vi "Settings Dialog.vi"(0 "Settings in":T9 {"Processing Settings"."Test Parameters"."Allowed Tolerance (%) FS" format="%#_4g"; "Acq Settings"."Config Settings"."Simulated Sensor Injection" scale=0.0..100.0}, 1 "Database in":refnum<queue>, 11 "error in (no error)":errorcluster) -> (3 "Database out":refnum<queue>, 4 "Settings out":T9 {"Processing Settings"."Test Parameters"."Allowed Tolerance (%) FS" format="%#_4g"; "Acq Settings"."Config Settings"."Simulated Sensor Injection" scale=0.0..100.0}, 6 "Measurements out":T7[](array[typedef]), 8 "UI Refresh Needed?":bool, 10 "Cancelled?":bool, 15 "error out":errorcluster)   [LabVIEW 2026, in "Settings.lvlib"]
doc: "Dialog for selecting user specified settings."
uses:
  Settings.lvlib
  controls/UI/Settings Cluster.ctl
  controls/UI/Acq Settings.ctl
  Acquisition/Instrument Specifications Configuration.ctl
  Acquisition/Instrument Specifications Cluster Configuration.ctl
  controls/UI/Measurement Role.ctl
  controls/UI/Config Settings.ctl
  Processing/Processing Settings.ctl
  controls/Messaging Payloads/Sensor CoreData.ctl
  controls/Messaging Payloads/Sensor CoreData Cluster.ctl
  controls/UI/Units Enum.ctl
  controls/UI/Signal Enum.ctl
  Processing/Test Parameters.ctl
  Processing/Test Parameters Cluster.ctl
  controls/UI/Test Sequence Context.ctl
  controls/UI/Direction.ctl
  controls/UI/Session Identfiers.ctl
  controls/UI/Test Sequence Settings.ctl
  controls/UI/Test Sequence State.ctl
  controls/UI/Test Sequence Enum.ctl
  controls/Controller/Stimulus Settings.ctl
  controls/Controller/Stimulus Outputs.ctl
  controls/Controller/Stimulus Output.ctl
  controls/Controller/Controller Core Data.ctl
  controls/Controller/Stimulus Output Configuration.ctl
  controls/Controller/Stimulus Role.ctl
  support/Architecture/Message Queue/Message Cluster.ctl
  controls/UI/Measurements Config.ctl
  controls/UI/Measurement Config.ctl
  controls/UI/Stimulus Outputs Display.ctl
  controls/UI/Stimulus Output Display.ctl
  controls/UI/Settings Refs.ctl
  controls/UI/UI List Type.ctl
  controls/UI/Data Entity.ctl
  Acquisition/Acquisition.lvlib
  support/Architecture/Message Queue/Message Queue.lvlib
  Processing/Processing_Engine.lvlib
panel:
  in  "STIMULUS OUTPUTS":T1
  out "INSTRUMENT CONFIGURATIONS":T4
  in  "MEASUREMENTS":T8
  in  "Operator":string(combo)
  in  "Cancel Button":bool
  in  "OK Button":bool
  # "Non visible portion of dialog (needed for connector pane)."
  # "* Database-configured values. Maintained by an Administrator."
  # "Physical Channel and Measurement Role are assigned in the Measurements section directly below."
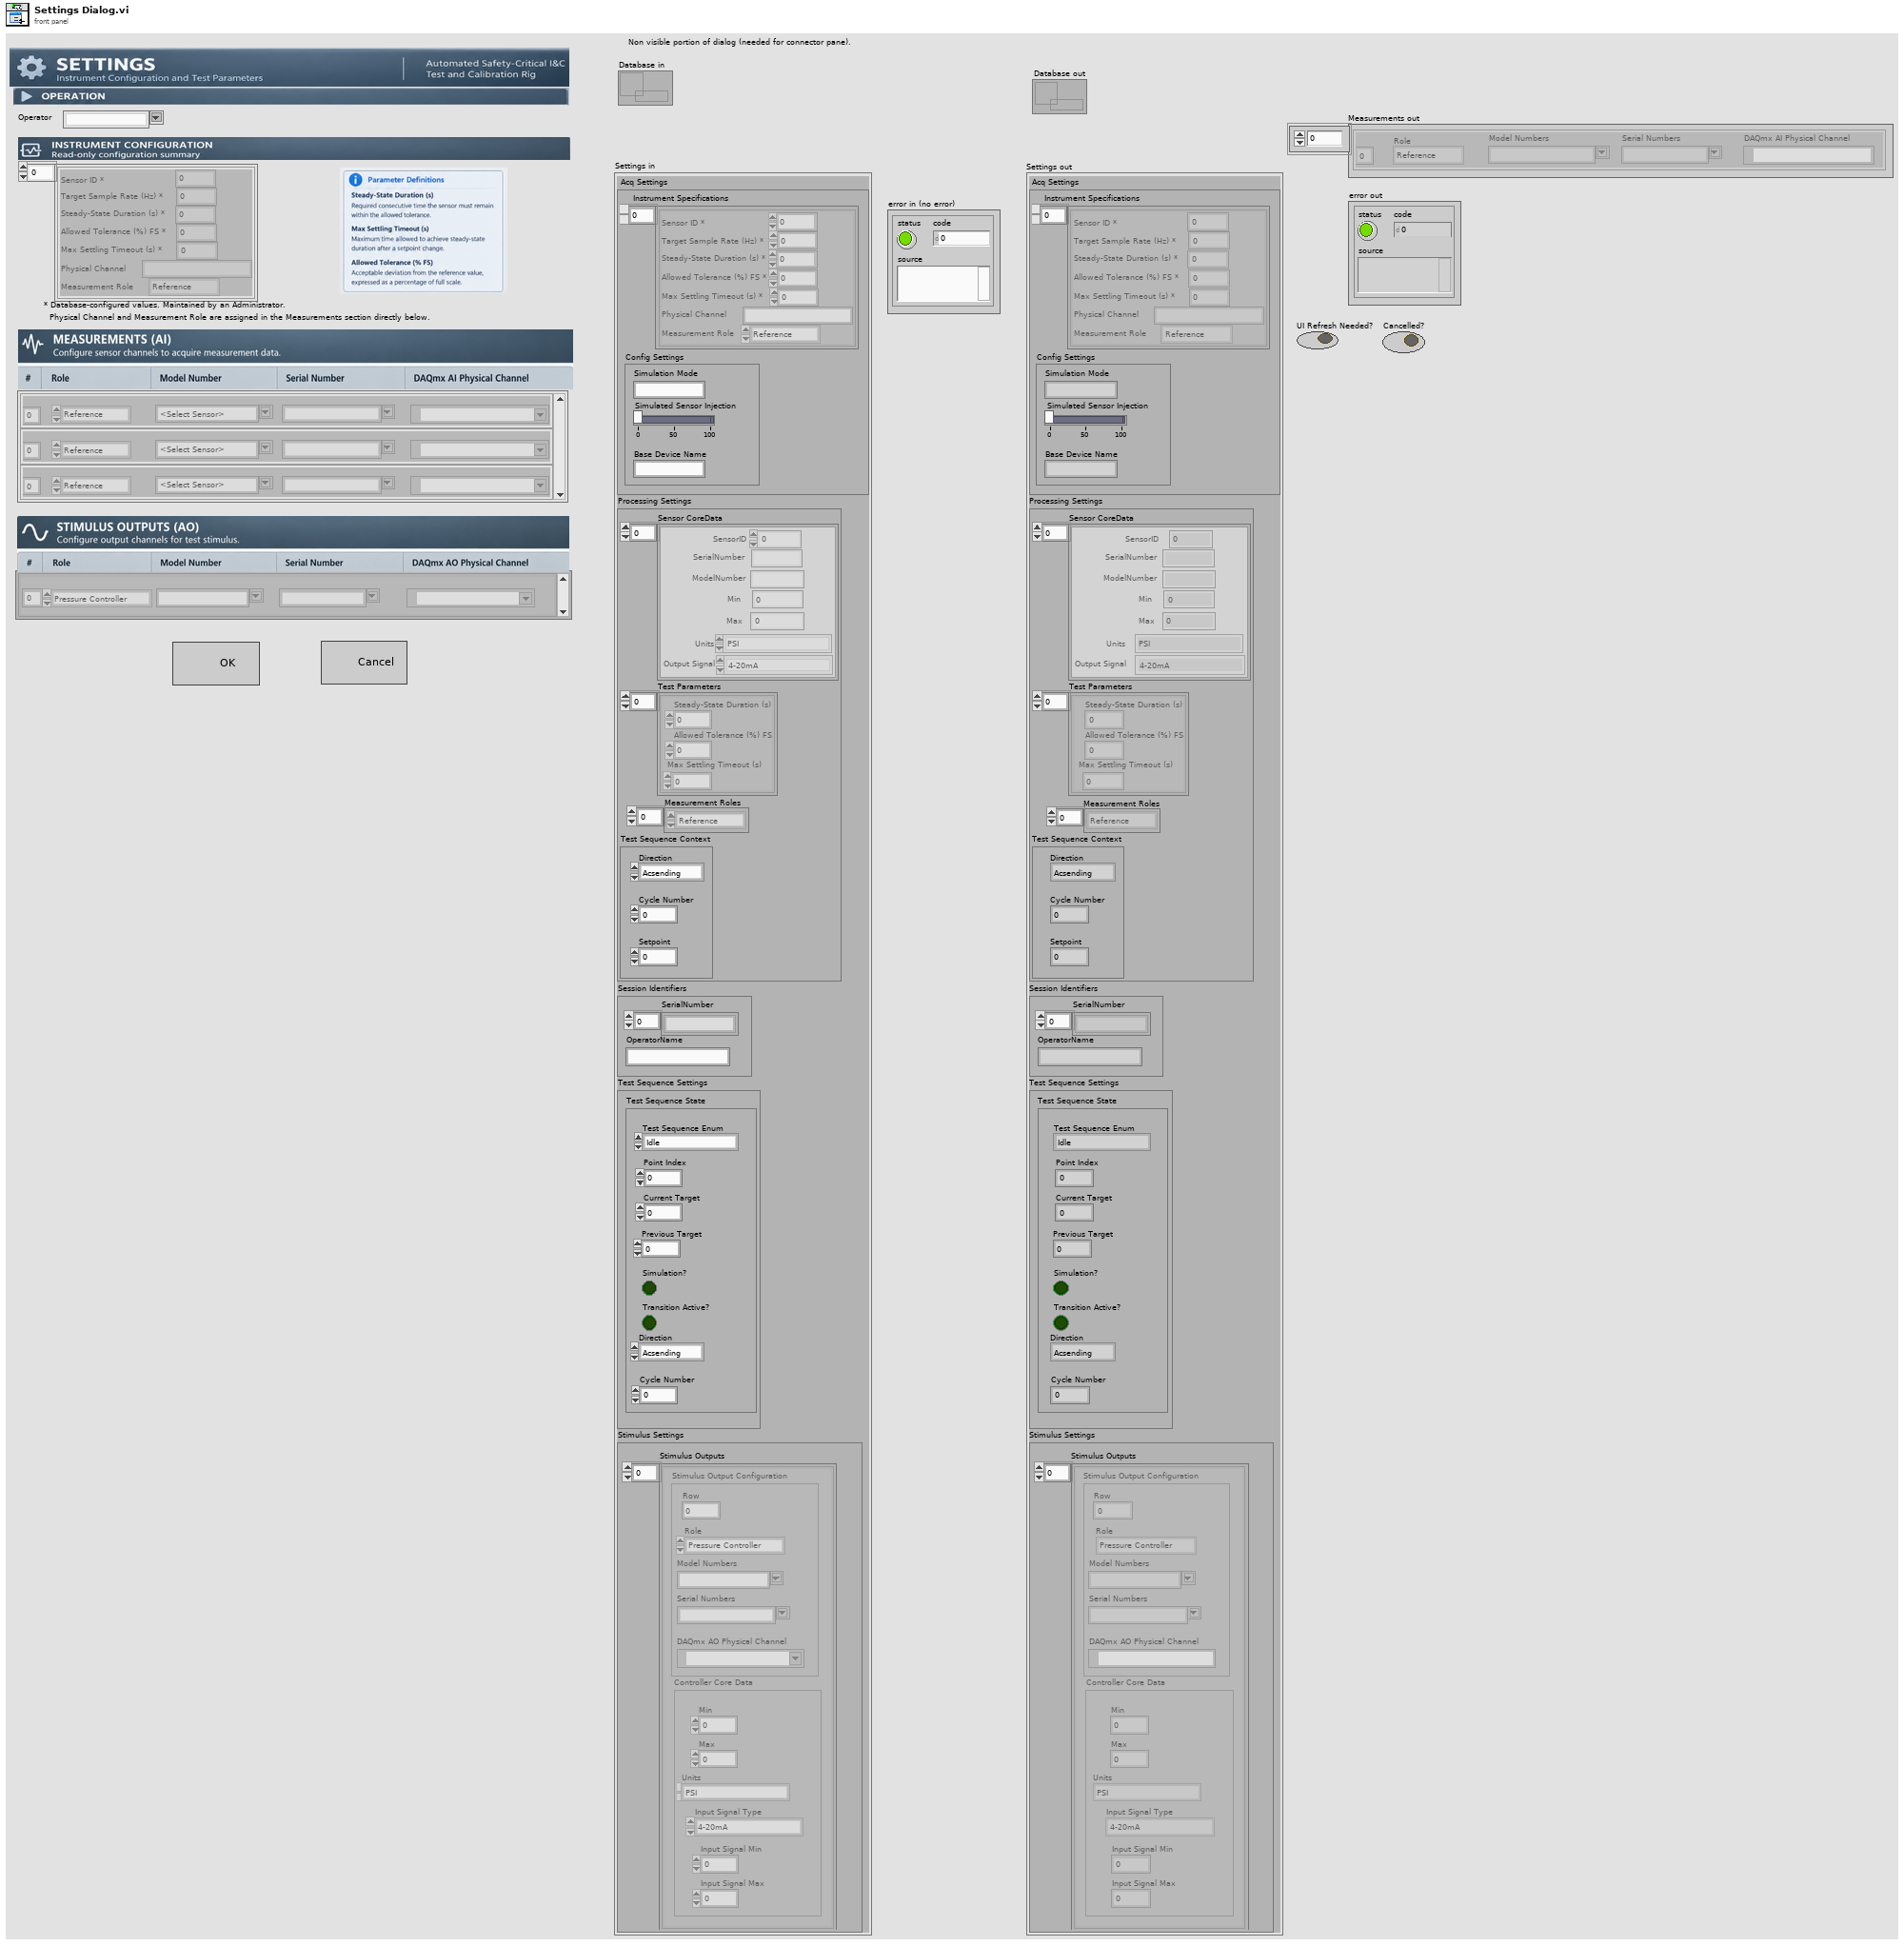
[diagram p1: front panel]
types:
  T1 = typedef "Settings.lvlib/Stimulus Outputs Display.ctl" = T2[]
  T2 = typedef "Settings.lvlib/Stimulus Output Display.ctl" = cluster{"DAQmx AO Physical Channel":tag, "Role":T3, "Model Numbers":string, "Serial Numbers":string, "Row":i32}
  T3 = typedef "Stimulus Role.ctl" = enum16{"Pressure Controller", "Temperature Controller"}
  T4 = typedef "Acquisition.lvlib/Instrument Specifications Configuration.ctl" = T5[]
  T5 = typedef "Acquisition.lvlib/Instrument Specifications Cluster Configuration.ctl" = cluster{"Sensor ID *":i32, "Target Sample Rate (Hz) *":dbl, "Steady-State Duration (s) *":i32, "Allowed Tolerance (%) FS *":dbl, "Max Settling Timeout (s) *":i32, "Physical Channel":string, "Measurement Role":T6}
  T6 = typedef "Settings.lvlib/Measurement Role.ctl" = enum16{"Reference", "UUT"}
  T7 = typedef "Measurement Config.ctl" = cluster{"DAQmx AI Physical Channel":tag, "Serial Numbers":string, "Model Numbers":string, "Role":T6, "Row":i32}
  T8 = typedef "Measurements Config.ctl" = T7[]
  T9 = typedef "Settings Cluster.ctl" = cluster{"Acq Settings":T10, "Processing Settings":T12, "Session Identifiers":T21, "Test Sequence Settings":T22, "Stimulus Settings":T25}
  T10 = typedef "Acq Settings.ctl" = cluster{"Instrument Specifications":T4, "Config Settings":T11}
  T11 = typedef "Config Settings.ctl" = cluster{"Simulated Sensor Injection":dbl, "Base Device Name":string, "Simulation Mode":string}
  T12 = typedef "Processing_Engine.lvlib/Processing Settings.ctl" = cluster{"Sensor CoreData":T13, "Test Parameters":T17, "Measurement Roles":T6[], "Test Sequence Context":T19}
  T13 = typedef "Sensor CoreData.ctl" = T14[]
  T14 = typedef "Settings.lvlib/Sensor CoreData Cluster.ctl" = cluster{"SerialNumber":string, "ModelNumber":string, "Min":dbl, "Max":dbl, "Units":T15, "Output Signal":T16, "SensorID":i32}
  T15 = typedef "Units Enum.ctl" = enum16{"PSI", "Deg C", "kPa", "GPM"}
  T16 = typedef "Signal Enum.ctl" = enum16{"4-20mA", "0-10V", "Thermocouple Type K"}
  T17 = typedef "Processing_Engine.lvlib/Test Parameters.ctl" = T18[]
  T18 = typedef "Settings.lvlib/Test Parameters Cluster.ctl" = cluster{"Steady-State Duration (s)":i32, "Allowed Tolerance (%) FS":dbl, "Max Settling Timeout (s)":i32}
  T19 = typedef "Settings.lvlib/Test Sequence Context.ctl" = cluster{"Direction":T20, "Cycle Number":i32, "Setpoint":dbl}
  T20 = typedef "Settings.lvlib/Direction.ctl" = enum16{"Acsending", "Descending"}
  T21 = typedef "Session Identfiers.ctl" = cluster{"SerialNumber":string[], "OperatorName":string}
  T22 = typedef "Test Sequence Settings.ctl" = cluster{"Test Sequence State":T23}
  T23 = typedef "Settings.lvlib/Test Sequence State.ctl" = cluster{"Test Sequence Enum":T24, "Point Index":i32, "Current Target":dbl, "Previous Target":dbl, "Simulation?":bool, "Direction":T20, "Transition Active?":bool, "Cycle Number":i32}
  T24 = typedef "Test Sequence Enum.ctl" = enum16{"Idle", "Start Point", "Point Complete", "Test Complete", "Abort Test", "Reset"}
  T25 = typedef "Settings.lvlib/Stimulus Settings.ctl" = cluster{"Stimulus Outputs":T26}
  T26 = typedef "Settings.lvlib/Stimulus Outputs.ctl" = T27[]
  T27 = typedef "Settings.lvlib/Stimulus Output.ctl" = cluster{"Controller Core Data":T28, "Stimulus Output Configuration":T29}
  T28 = typedef "Settings.lvlib/Controller Core Data.ctl" = cluster{"Min":dbl, "Max":dbl, "Units":T15, "Input Signal Type":T16, "Input Signal Min":dbl, "Input Signal Max":dbl}
  T29 = typedef "Settings.lvlib/Stimulus Output Configuration.ctl" = cluster{"DAQmx AO Physical Channel":tag, "Role":T3, "Model Numbers":string, "Serial Numbers":string, "Row":i32}
  T30 = typedef "Settings Refs.ctl" = cluster{"Serial Numbers Ref":refnum<vi>, "Logging Ref":refnum<vi>, "Model Numbers Ref":refnum<vi>, "OK Ref":refnum<vi>, "Instrument Specifications Cluster Ref":refnum<vi>, "Instrument Specifications Ref":refnum<vi>, "Measurements Ref":refnum<vi>, "Stimulus Outputs Ref":refnum<vi>}
  T31 = typedef "Settings.lvlib/Data Entity.ctl" = enum16{"Measurement", "Controller", " Test Configuration"}
  T32 = enum8{"Enabled", "Disabled", "Disabled and Grayed Out"}
  T33 = typedef "UI List Type.ctl" = enum16{"Model Numbers", "Serial Numbers", "Operators", "Calibration Points", "Start Run Times"}
  T34 = typedef "LVPoint32TypeDef.ctl" = cluster{"Horizontal":i32, "Vertical":i32}
  T35 = typedef "MSG FetchConfiguration Payload.ctl" = cluster{"Serial Numbers":string[], "Hardware Settings Cluster":T5}
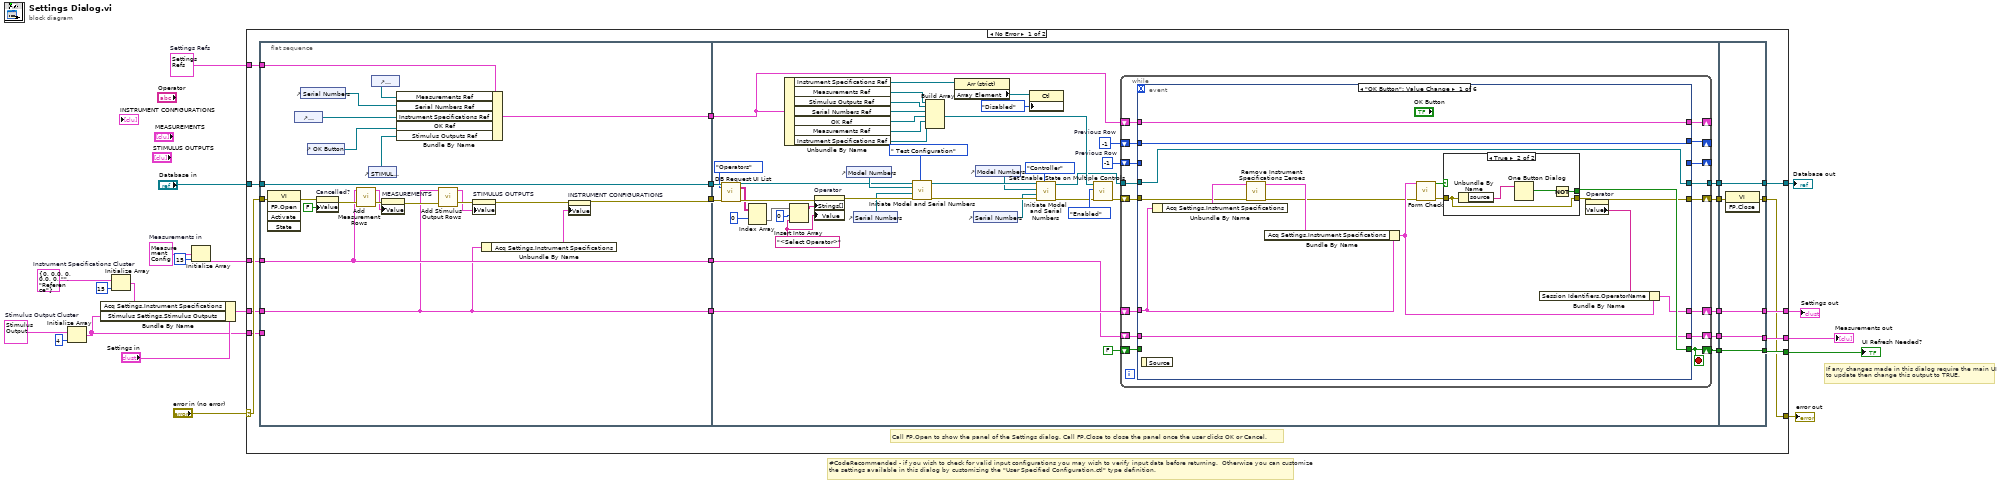
[diagram p0: block diagram]
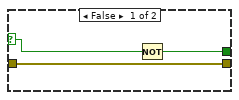
[diagram p2: hidden frame]
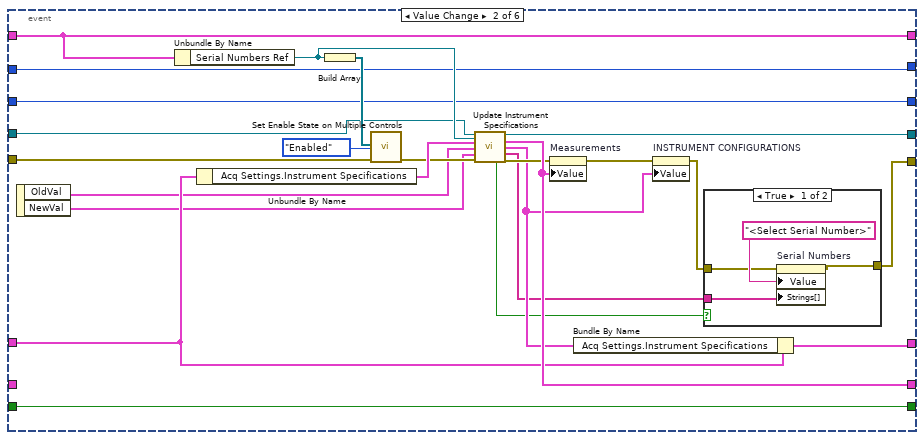
[diagram p3: hidden frame]
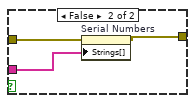
[diagram p4: hidden frame]
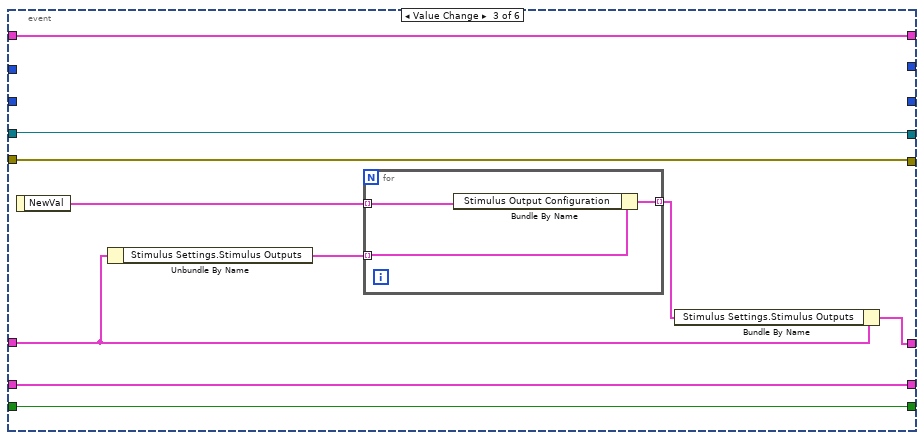
[diagram p5: hidden frame]
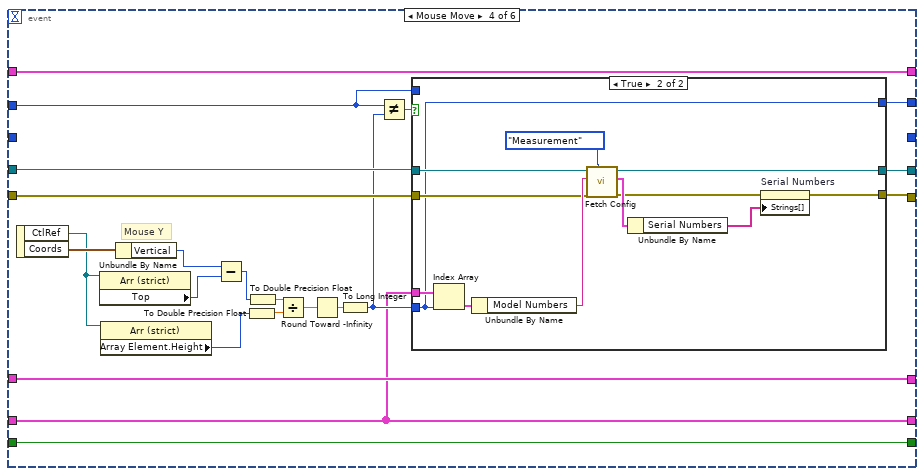
[diagram p6: hidden frame]
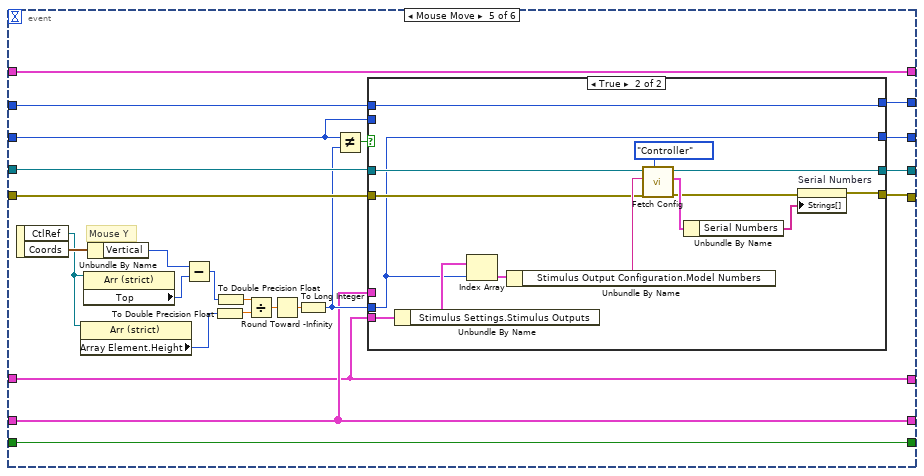
[diagram p8: hidden frame]
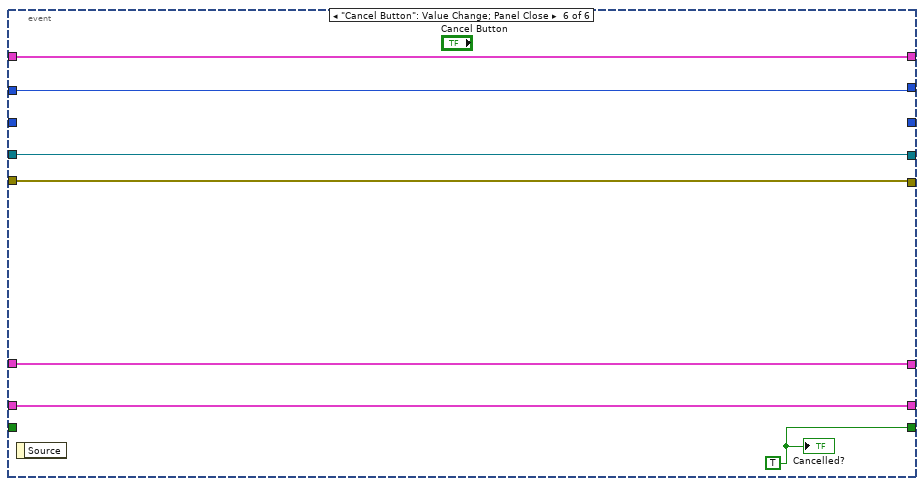
[diagram p10: hidden frame]
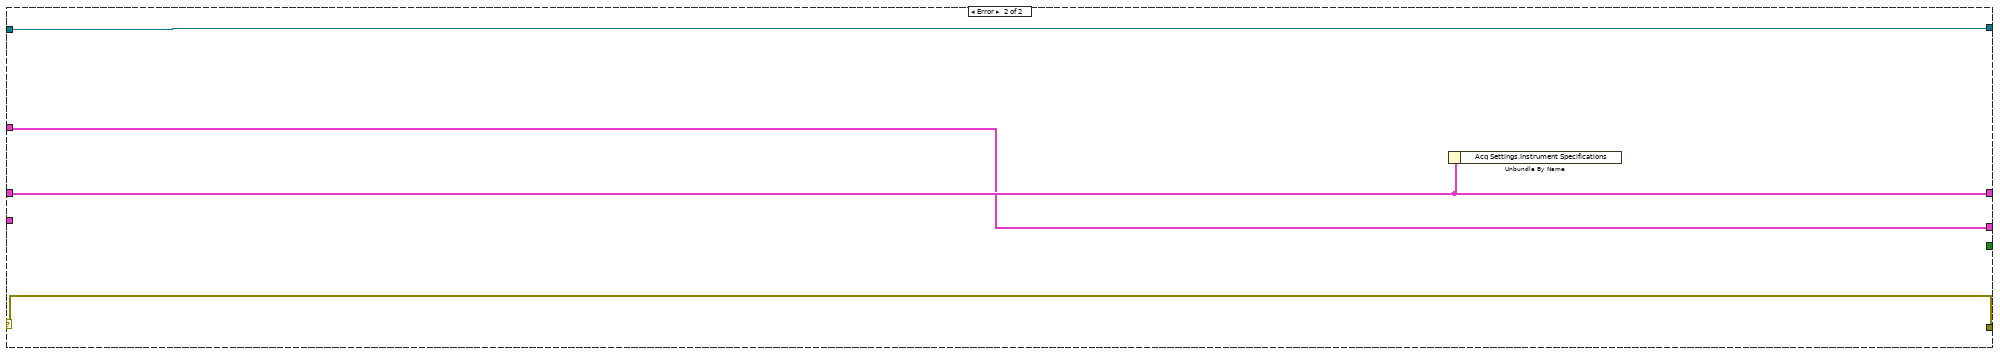
[diagram p11: hidden frame]
diagram:
  w2 = T27 {"Controller Core Data"={"Min"=0.0, "Max"=0.0, "Units"=enum."PSI", "Input Signal Type"=enum."4-20mA", "Input Signal Min"=0.0, "Input Signal Max"=0.0}, "Stimulus Output Configuration"={"DAQmx AO Physical Channel"="", "Role"=enum."Pressure Controller", "Model Numbers"="", "Serial Numbers"="", "Row"=0}}  # Stimulus Output Cluster
  w8 = T5 {"Sensor ID *"=0, "Target Sample Rate (Hz) *"=0.0, "Steady-State Duration (s) *"=0, "Allowed Tolerance (%) FS *"=0.0, "Max Settling Timeout (s) *"=0, "Physical Channel"="", "Measurement Role"=enum."Reference"}  # Instrument Specifications Cluster
  w12 = T7 {"DAQmx AI Physical Channel"="", "Serial Numbers"="", "Model Numbers"="<Select Sensor>", "Role"=enum."Reference", "Row"=0}  # Measurements in
  w16 = T30 {"Serial Numbers Ref"=refnum, "Logging Ref"=refnum, "Model Numbers Ref"=refnum, "OK Ref"=refnum, "Instrument Specifications Cluster Ref"=refnum, "Instrument Specifications Ref"=refnum, "Measurements Ref"=refnum, "Stimulus Outputs Ref"=refnum}  # Settings Refs
  # "If any changes made in this dialog require the main UI to update then change this output to TRUE."
  # "#CodeRecommended - if you wish to check for valid input configurations you may wish to verify input data before returning.  Otherwise you can customize the settings available in this dialog by customizing the \"User Specified Configuration.ctl\" type definition."
  n1 = Initialize Array(w2, 4 ("dimension size")) -> (w1:T27[])
  n2 = Initialize Array(w8, 15 ("dimension size")) -> (w7:T5[])
  n3 = Bundle By Name(cluster="Settings in", "Acq Settings.Instrument Specifications"=w7, "Stimulus Settings.Stimulus Outputs"=w1) -> (w6:T9)
  n4 = Initialize Array(w12, 15 ("dimension size")) -> (w10:T7[])
  n5 = case shown="No Error" "error in (no error)" {
    selector: "error in (no error)" -> [w33 w287]
    tunnel: [w20 w287] -> w18
    tunnel: [w28 _] -> w17
    tunnel: "Database in" -> [w38 w285]
    tunnel: w16 -> [w34 _]
    tunnel: [w29 w286] -> w15
    tunnel: w6 -> [w31 w286]
    tunnel: [w26 w285] -> w14
    tunnel: w10 -> [w25 w284]
    tunnel: [w22 w284] -> w13
    tunnel: w1 -> [w21 _]
    frame No Error {
      # "Call FP.Open to show the panel of the Settings dialog. Call FP.Close to close the panel once the user clicks OK or Cancel."
      n6 = flat-sequence {
        tunnel: w38 -> [w61]
        tunnel: [w43] -> w36
        tunnel: w33 -> [w62]
        tunnel: [w61] -> w35
        tunnel: w34 -> [w58]
        tunnel: [w60] -> w32
        tunnel: w31 -> [w42]
        tunnel: [w42] -> w30
        tunnel: w25 -> [w45]
        tunnel: [w45] -> w24
        tunnel: w21 -> [_]
        tunnel: [w107] -> w40
        tunnel: [w106] -> w39
        tunnel: w36 -> [w99]
        tunnel: [w105] -> w37
        tunnel: w35 -> [w100]
        tunnel: w32 -> [w102]
        tunnel: w30 -> [w101]
        tunnel: [w93] -> w27
        tunnel: w24 -> [w89]
        tunnel: [w92] -> w23
        tunnel: [w283] -> w29
        tunnel: w40 -> [w280]
        tunnel: w39 -> [w283]
        tunnel: w37 -> [w282]
        tunnel: [w281] -> w20
        tunnel: [w280] -> w28
        tunnel: w27 -> [w279]
        tunnel: [w279] -> w26
        tunnel: w23 -> [w278]
        tunnel: [w278] -> w22
        frame #0 {
          n7 = invoke class="VI" method="FP.Open"(error in=w62) -> (error out=w57:errorcluster)  [unwired: 4 in, 4 out]
          n8 = control-ref of="INSTRUMENT CONFIGURATIONS"() -> (w52:refnum<vi>)
          n9 = control-ref of="Serial Numbers"() -> (w55:refnum<vi>)
          n10 = control-ref of="OK Button"() -> (w59:refnum<vi>)
          n11 = property on="Cancelled?" class="Bool (strict)"(error in=w57, "Value"=FALSE ("Cancelled?")) -> (error out=w51:errorcluster)  [unwired: 1 in, 1 out]
          n12 = call "Add Measurement Rows.vi"("error in (no error)"=w51, "Measurements in"=w45) -> ("error out"=w50:errorcluster, "Measurements out"=w49:T8)  [unwired: 8 in]
          n13 = control-ref of="STIMULUS OUTPUTS"() -> (w53:refnum<vi>)
          n14 = control-ref of="MEASUREMENTS"() -> (w54:refnum<vi>)
          n15 = property on="MEASUREMENTS" class="Arr (strict)"(error in=w50, "Value"=w49) -> (error out=w48:errorcluster)  [unwired: 1 in, 1 out]
          n16 = Bundle By Name(cluster=w58, "Measurements Ref"=w54, "Serial Numbers Ref"=w55, "Instrument Specifications Ref"=w52, "OK Ref"=w59, "Stimulus Outputs Ref"=w53) -> (w60:T30)
          n17 = call "Add Stimulus Output Rows.vi"("error in (no error)"=w48, "Settings"=w42) -> ("error out"=w47:errorcluster, "Stimulus Outputs"=w46:T1)  [unwired: 8 in]
          n18 = property on="STIMULUS OUTPUTS" class="Arr (strict)"(error in=w47, "Value"=w46) -> (error out=w44:errorcluster)  [unwired: 1 in, 1 out]
          n19 = Unbundle By Name(w42) -> ("Acq Settings.Instrument Specifications"=w41:T4)
          n20 = property on="INSTRUMENT CONFIGURATIONS" class="Arr (strict)"(error in=w44, "Value"=w41) -> (error out=w43:errorcluster)  [unwired: 1 in, 1 out]
        }
        frame #1 {
          w66 = -1  # Previous Row
          w90 = -1  # Previous Row
          w94 = "<Select Operator>"
          n21 = call "DB Request UI List.vi"("Database in"=w100, "UI List Type"=UI_List_Type."Operators", "error in (no error)"=w99) -> ("Database out"=w76:refnum<queue>, "Results"=w65:string[][], "error out"=w96:errorcluster)  [unwired: 14 in]
          n22 = Index Array(array=w65, index (row)=0 ("index")) -> (element=w63:string[])  [unwired: 1 in]
          n23 = Unbundle By Name(w102) -> ("Instrument Specifications Ref"=w81:refnum<vi>, "Measurements Ref"=w85:refnum<vi>, "Stimulus Outputs Ref"=w87:refnum<vi>, "Serial Numbers Ref"=w86:refnum<vi>, "OK Ref"=w83:refnum<vi>, "Measurements Ref"=w84:refnum<vi>, "Instrument Specifications Ref"=w82:refnum<vi>)
          n24 = Insert Into Array(array=w63, index=0, new element=w94) -> (w97:string[])
          n25 = property on="Operator" class="CmbBox"(error in=w96, "Strings[]"=w97, "Value"=w94) -> (error out=w95:errorcluster)  [unwired: 1 in, 1 out]
          n26 = control-ref of="Model Numbers"() -> (w77:refnum<vi>)
          n27 = control-ref of="Serial Numbers"() -> (w75:refnum<vi>)
          n28 = call "Initiate Model and Serial Numbers.vi"("UI Device Type"=Data_Entity." Test Configuration", "error in (no error)"=w95, "Serial CmbBox Ref"=w75, "Model CmbBox Ref"=w77, "Database in"=w76) -> ("error out"=w74:errorcluster, "Database out"=w72:refnum<queue>)  [unwired: 5 in]
          n29 = Build Array(w85, w87, w86, w83, w84, w82) -> (w103:refnum<vi>[])
          n30 = property class="Arr (strict)"(reference=w81) -> ("Array Element"=w80:refnum<vi>)  [unwired: 1 in, 2 out]
          n31 = control-ref of="Serial Numbers"() -> (w67:refnum<vi>)
          n32 = control-ref of="Model Numbers"() -> (w68:refnum<vi>)
          n33 = property class="Ctl"(reference=w80, "DisabledEnum"=T32."Disabled" ("Disabled")) -> ()  [unwired: 1 in, 2 out]
          n34 = call "Initiate Model and Serial Numbers.vi"("UI Device Type"=Data_Entity."Controller", "error in (no error)"=w74, "Serial CmbBox Ref"=w67, "Model CmbBox Ref"=w68, "Database in"=w72) -> ("error out"=w73:errorcluster, "Database out"=w71:refnum<queue>)  [unwired: 5 in]
          n35 = call "Set Enable State on Multiple Controls.vi"("Controls"=w103, "Disabled"=T32."Enabled", "error in (no error)"=w73) -> ("error out"=w78:errorcluster)  [unwired: 7 in]
          n36 = while {
            tunnel: w71 -> [w119]
            shift-right: [w123] -> w106
            shift-left: w101 -> [w122]
            shift-right: [w121] -> w105
            shift-left: w78 -> [w120]
            shift-right: [w115] -> w107
            shift-left: FALSE ("UI Refresh Needed?") -> [w118]
            shift-right: [w116] -> _
            shift-left: w102 -> [w117]
            tunnel: [w114] -> w93
            shift-right: [w110] -> _
            shift-left: w90 -> [w111]
            shift-right: [w113] -> w92
            shift-left: w89 -> [w112]
            shift-right: [w108] -> _
            shift-left: w66 -> [w109]
            stop <- w115 stop-if-true
            n37 = event shown="[0] \"OK Button\": Value Change" {
              selector: _ -> [_ _ _ _ _ _]
              dyn-events: _ -> [_ _ _ _ _ _]
              timeout: _ -> [_ _ _ _ _ _]
              tunnel: [w134 w165 w183 w213 w230 w277] -> w123
              tunnel: w122 -> [w127 w166 w185 w213 w230 w277]
              tunnel: [w138 w171 w181 w192 w233 w275] -> w115
              tunnel: w120 -> [w125 w164 w180 w200 w240 w276]
              tunnel: [w132 w155 w180 w194 w235 w276] -> w121
              tunnel: w119 -> [w133 w150 w187 w201 w241 w273]
              tunnel: w118 -> [_ w171 w181 w192 w233 _]
              tunnel: w117 -> [w137 w152 w188 w212 w252 w274]
              tunnel: [w137 w152 w188 w212 w252 w274] -> w116
              tunnel: [w133 w149 w187 w199 w239 w273] -> w114
              tunnel: [w131 w170 w182 w193 w234 w272] -> w113
              tunnel: w112 -> [w131 _ w182 w193 w234 w272]
              tunnel: w111 -> [w130 w153 _ w195 w236 w271]
              tunnel: [w130 w153 _ w196 w237 w271] -> w110
              tunnel: w109 -> [_ w148 _ _ w231 _]
              tunnel: [_ w148 _ _ w229 _] -> w108
              event "OK Button": Value Change {
                n38 = event-data() -> ()  [unwired: 1 in, 1 out]
                n39 = Unbundle By Name(w127) -> ("Acq Settings.Instrument Specifications"=w129:T4)
                n40 = call "Remove Instrument Specifications Zeroes.vi"("error in (no error)"=w125, "INSTRUMENT CONFIGURATIONS in"=w129) -> ("error out"=w124:errorcluster, "INSTRUMENT CONFIGURATIONS out"=w128:T4)  [unwired: 8 in]
                n41 = Bundle By Name(cluster=w127, "Acq Settings.Instrument Specifications"=w128) -> (w126:T9)
                n42 = call "Form Check.vi"("error in (no error)"=w124, "Config in"=w126) -> ("error out"=w139:errorcluster, "Form Error?"=w140:bool)  [unwired: 8 in]
                n43 = case shown="True" w140 {
                  selector: w140 -> [w142 _]
                  tunnel: w139 -> [w141 w144]
                  tunnel: [w143 w145] -> w138
                  tunnel: [w141 w144] -> w136
                  frame False {
                    n44 = Not(x=w142) -> (.not. x?=w143:bool)
                  }
                  frame True {
                    n45 = Unbundle By Name(w144) -> ("source"=w147:string)
                    n46 = One Button Dialog(message=w147) -> (true=w146:bool)  [unwired: 1 in]
                    n47 = Not(x=w146) -> (.not. x?=w145:bool)
                  }
                }
                n48 = property on="Operator" class="CmbBox"(error in=w136) -> (error out=w132:errorcluster, "Value"=w135:string)  [unwired: 1 in, 1 out]
                n49 = Bundle By Name(cluster=w126, "Session Identifiers.OperatorName"=w135) -> (w134:T9)
              }
              event Value Change {
                n50 = event-data() -> ("OldVal"=w162:T8, "NewVal"=w161:T8)  [unwired: 1 in]
                n51 = Unbundle By Name(w152) -> ("Serial Numbers Ref"=w160:refnum<vi>)
                n52 = Unbundle By Name(w166) -> ("Acq Settings.Instrument Specifications"=w167:T4)
                n53 = Build Array(w160) -> (w159:refnum<vi>[])
                n54 = call "Set Enable State on Multiple Controls.vi"("Controls"=w159, "Disabled"=T32."Enabled", "error in (no error)"=w164) -> ("error out"=w163:errorcluster)  [unwired: 7 in]
                n55 = call "Update Instrument Specifications.vi"("Queue in"=w150, "Serial Numbers Ref"=w160, "Instrument Specifications in"=w167, "OldVal"=w162, "NewVal"=w161, "error in (no error)"=w163) -> ("Queue out"=w149:refnum<queue>, "Measurements"=w170:T7[], "Instrument Specifications out"=w158:T4, "Serial Numbers"=w154:string[], "Serial Number Header?"=w157:bool, "error out"=w169:errorcluster)  [unwired: 4 in]
                n56 = property on="Measurements" class="Arr (strict)"(error in=w169, "Value"=w170) -> (error out=w168:errorcluster)  [unwired: 1 in, 1 out]
                n57 = Bundle By Name(cluster=w166, "Acq Settings.Instrument Specifications"=w158) -> (w165:T9)
                n58 = property on="INSTRUMENT CONFIGURATIONS" class="Arr (strict)"(error in=w168, "Value"=w158) -> (error out=w156:errorcluster)  [unwired: 1 in, 1 out]
                n59 = case shown="True" w157 {
                  tunnel: w156 -> [w174 w178]
                  tunnel: [w173 w177] -> w155
                  tunnel: w154 -> [w172 w176]
                  frame True {
                    n60 = property on="Serial Numbers" class="CmbBox"(error in=w174, "Value"="<Select Serial Number>", "Strings[]"=w172) -> (error out=w173:errorcluster)  [unwired: 1 in, 1 out]
                  }
                  frame False {
                    n61 = property on="Serial Numbers" class="CmbBox"(error in=w178, "Strings[]"=w176) -> (error out=w177:errorcluster)  [unwired: 1 in, 1 out]
                  }
                }
              }
              event Value Change {
                n62 = event-data() -> ("NewVal"=w179:T1)  [unwired: 1 in]
                n63 = Unbundle By Name(w185) -> ("Stimulus Settings.Stimulus Outputs"=w186:T26)
                n64 = for {
                  tunnel: w186 -> [w191] mode=indexing
                  tunnel: w179 -> [w189] mode=indexing
                  tunnel: [w190] -> w184 mode=indexing
                  n65 = Bundle By Name(cluster=w191, "Stimulus Output Configuration"=w189) -> (w190:T27)
                }
                n66 = Bundle By Name(cluster=w185, "Stimulus Settings.Stimulus Outputs"=w184) -> (w183:T9)
              }
              event Mouse Move {
                # "Mouse Y"
                n67 = event-data() -> ("CtlRef"=w208:refnum<vi>, "Coords"=w211:T34)  [unwired: 1 in]
                n68 = property class="Arr (strict)"(reference=w208) -> ("Top"=w209:i32)  [unwired: 1 in, 2 out]
                n69 = property class="Arr (strict)"(reference=w208) -> ("Array Element.Height"=w205:u32)  [unwired: 1 in, 2 out]
                n70 = Unbundle By Name(w211) -> ("Vertical"=w210:i32)
                n71 = Subtract(x=w210, y=w209) -> (x-y=w207:i32)
                n72 = To Double Precision Float(number=w205) -> (double precision float=w204:dbl)
                n73 = To Double Precision Float(number=w207) -> (double precision float=w206:dbl)
                n74 = Divide(x=w206, y=w204) -> (x/y=w203:dbl)
                n75 = Round Toward -Infinity(1:w203) -> (0:w202:dbl)
                n76 = To Long Integer(number=w202) -> (32bit integer=w198:i32)
                n77 = Not Equal?(x=w195, y=w198) -> (x != y?=w197:bool)
                n78 = case shown="True" w197 {
                  tunnel: w193 -> [_ w228]
                  tunnel: w201 -> [w215 w225]
                  tunnel: w200 -> [w214 w224]
                  tunnel: [w215 w223] -> w199
                  tunnel: [w214 w219] -> w194
                  tunnel: w198 -> [_ w221]
                  tunnel: [w216 w221] -> w196
                  tunnel: w195 -> [w216 _]
                  frame False {
                  }
                  frame True {
                    n79 = Index Array(array=w228, index=w221) -> (element=w227:T7)
                    n80 = Unbundle By Name(w227) -> ("Model Numbers"=w226:string)
                    n81 = call "Fetch Config.vi"("UI Device Type"=Data_Entity."Measurement", "error in (no error)"=w224, "ModelNumber"=w226, "Database in"=w225) -> ("error out"=w220:errorcluster, "Model Details Payload"=w222:T35, "Database out"=w223:refnum<queue>)  [unwired: 5 in]
                    n82 = Unbundle By Name(w222) -> ("Serial Numbers"=w218:string[])
                    n83 = property on="Serial Numbers" class="CmbBox"(error in=w220, "Strings[]"=w218) -> (error out=w219:errorcluster)  [unwired: 1 in, 1 out]
                  }
                }
              }
              event Mouse Move {
                # "Mouse Y"
                n84 = event-data() -> ("CtlRef"=w248:refnum<vi>, "Coords"=w251:T34)  [unwired: 1 in]
                n85 = property class="Arr (strict)"(reference=w248) -> ("Array Element.Height"=w245:u32)  [unwired: 1 in, 2 out]
                n86 = property class="Arr (strict)"(reference=w248) -> ("Top"=w249:i32)  [unwired: 1 in, 2 out]
                n87 = Unbundle By Name(w251) -> ("Vertical"=w250:i32)
                n88 = Subtract(x=w250, y=w249) -> (x-y=w247:i32)
                n89 = To Double Precision Float(number=w245) -> (double precision float=w244:dbl)
                n90 = To Double Precision Float(number=w247) -> (double precision float=w246:dbl)
                n91 = Divide(x=w246, y=w244) -> (x/y=w243:dbl)
                n92 = Round Toward -Infinity(1:w243) -> (0:w242:dbl)
                n93 = To Long Integer(number=w242) -> (32bit integer=w238:i32)
                n94 = Not Equal?(x=w231, y=w238) -> (x != y?=w232:bool)
                n95 = case shown="True" w232 {
                  tunnel: w234 -> [_ _]
                  tunnel: w241 -> [w255 w269]
                  tunnel: w240 -> [w254 w268]
                  tunnel: [w255 w267] -> w239
                  tunnel: [w254 w258] -> w235
                  tunnel: w238 -> [_ w261]
                  tunnel: [w256 w260] -> w237
                  tunnel: w236 -> [w256 w260]
                  tunnel: w231 -> [w253 _]
                  tunnel: w230 -> [_ w264]
                  tunnel: [w253 w261] -> w229
                  frame False {
                  }
                  frame True {
                    n96 = Unbundle By Name(w264) -> ("Stimulus Settings.Stimulus Outputs"=w263:T26)
                    n97 = Index Array(array=w263, index=w261) -> (element=w262:T27)
                    n98 = Unbundle By Name(w262) -> ("Stimulus Output Configuration.Model Numbers"=w270:string)
                    n99 = call "Fetch Config.vi"("UI Device Type"=Data_Entity."Controller", "error in (no error)"=w268, "ModelNumber"=w270, "Database in"=w269) -> ("error out"=w259:errorcluster, "Model Details Payload"=w266:T35, "Database out"=w267:refnum<queue>)  [unwired: 5 in]
                    n100 = Unbundle By Name(w266) -> ("Serial Numbers"=w257:string[])
                    n101 = property on="Serial Numbers" class="CmbBox"(error in=w259, "Strings[]"=w257) -> (error out=w258:errorcluster)  [unwired: 1 in, 1 out]
                  }
                }
              }
              event "Cancel Button": Value Change; Panel Close {
                w275 = TRUE ("UI Refresh Needed?")
                n102 = event-data() -> ()  [unwired: 1 in, 1 out]
                "Cancelled?" <- w275
              }
            }
          }
        }
        frame #2 {
          n103 = invoke class="VI" method="FP.Close"(error in=w282) -> (error out=w281:errorcluster)  [unwired: 2 in, 2 out]
        }
      }
    }
    frame Error {
      n104 = Unbundle By Name(w286) -> ()  [unwired: 1 out]
    }
  }
  "UI Refresh Needed?" <- w17
  "error out" <- w18
  "Settings out" <- w15
  "Database out" <- w14
  "Measurements out" <- w13
